vi "test.vi"() -> ()   [LabVIEW 2023]
uses:
  LeCroy HDO4000A/LeCroy HDO4000A.lvclass
  Configurations/Fetch Display CFG/Fetch Display CFG.lvclass
  D:/git/LeCroy-HDO4000A-LabVIEW/Configurations/HDO4000A Base CFG/HDO4000A Base CFG.lvclass
  D:/git/HAL/Scope VISA/Configuration/Scope VISA CFG.lvclass
  D:/git/HAL/Configuration Base/Configuration Base.lvclass
  D:/git/HAL/Interfaces/IConfigure/IConfigure.lvclass
  D:/git/HAL/Interfaces/IConfigure Scope/IConfigure Scope.lvclass
  D:/git/LeCroy-HDO4000A-LabVIEW/Configurations/Fetch Display CFG/Fetch Display CFG.lvclass
panel:
  out "Last Waveform Mean":dbl
  out "Last Waveform":waveform(dbl)(graph)
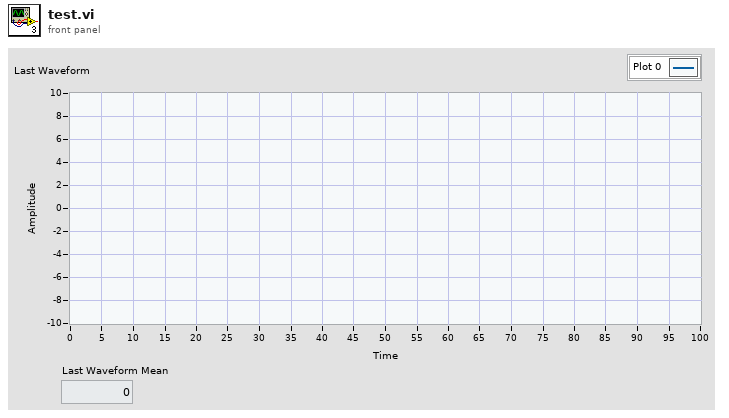
[diagram p1: front panel]
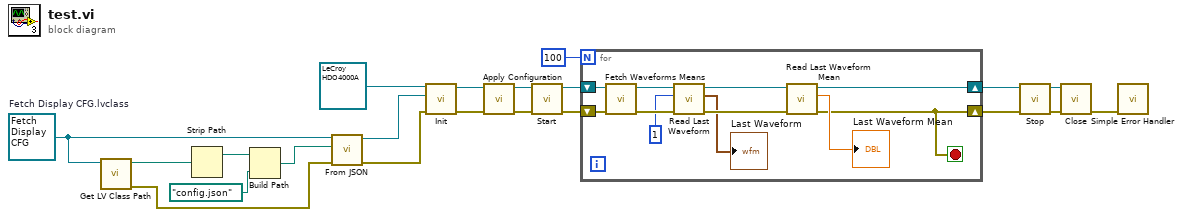
[diagram p0: block diagram]
diagram:
  w15 = refnum<class "Fetch Display CFG.lvclass"> refnum  # Fetch Display CFG.lvclass
  n1 = call <vilib>:"Get LV Class Path.vi"("object"=w15) -> ("error out"=w11:errorcluster, "class path"=w16:path)  [unwired: 9 in]
  n2 = Strip Path(path=w16) -> (stripped path=w14:path)  [unwired: 1 out]
  n3 = Build Path(base path=w14, name or relative path=path "config.json") -> (appended path=w12:path)
  n4 = call-dynamic "From JSON.vi"("error in (no error)"=w11, "JSON Config"=w12, "object in"=w15) -> ("error out"=w17:errorcluster, "object out"=w21:refnum<class "Fetch Display CFG.lvclass">)  [unwired: 7 in]
  n5 = call-dynamic "Init.vi"("Error In"=w17, "HAL.lvlib:IConfigure"=w21, "object in"=refnum<class "LeCroy HDO4000A.lvclass"> refnum ("LeCroy HDO4000A.lvclass")) -> ("Error Out"=w6:errorcluster, "object out"=w5:refnum<class "LeCroy HDO4000A.lvclass">)  [unwired: 7 in]
  n6 = call-dynamic "Apply Configuration.vi"("error in"=w6, "Scope Base in"=w5) -> ("error out"=w7:errorcluster, "Scope Base out"=w4:refnum<class "LeCroy HDO4000A.lvclass">)  [unwired: 8 in]
  n7 = call-dynamic "Start.vi"("Error In"=w7, "object in"=w4) -> ("Error Out"=w19:errorcluster, "object out"=w10:refnum<class "LeCroy HDO4000A.lvclass">)  [unwired: 8 in]
  n8 = for {
    N: 100 -> [_]
    shift-right: [w22] -> w9
    shift-left: w19 -> [w32]
    shift-right: [w23] -> w8
    shift-left: w10 -> [w31]
    stop <- w22 stop-if-true
    n9 = call-dynamic "Fetch Waveforms Means.vi"("error in"=w32, "Scope Base in"=w31) -> ("error out"=w28:errorcluster, "Scope Base out"=w29:refnum<class "LeCroy HDO4000A.lvclass">)  [unwired: 8 in]
    n10 = call-dynamic "Read Last Waveform.vi"("error in (no error)"=w28, "Channel"=u8 1, "Scope Base in"=w29) -> ("error out"=w27:errorcluster, "Last Waveform"=→"Last Waveform":waveform(dbl), "Scope Base out"=w30:refnum<class "LeCroy HDO4000A.lvclass">)  [unwired: 6 in]
    n11 = call-dynamic "Read Last Waveform Mean.vi"("error in (no error)"=w27, "Scope Base in"=w30) -> ("error out"=w22:errorcluster, "Waveform Mean"=→"Last Waveform Mean":dbl, "Scope Base out"=w23:refnum<class "LeCroy HDO4000A.lvclass">)  [unwired: 7 in]
  }
  n12 = call-dynamic "Stop.vi"("Error In"=w9, "object in"=w8) -> ("Error Out"=w3:errorcluster, "object out"=w2:refnum<class "LeCroy HDO4000A.lvclass">)  [unwired: 8 in]
  n13 = call-dynamic "Close.vi"("Error In"=w3, "object in"=w2) -> ("Error Out"=w1:errorcluster)  [unwired: 8 in, 1 out]
  n14 = call <vilib>:"Simple Error Handler.vi"("error in (no error)"=w1) -> ()  [unwired: 4 in, 5 out]
